vi "awg_memReplay.vi"(6 "reset":bool, 7 "memSelector":refnum<k21>, 9 "periodic":bool, 10 "clocks":T2, 11 "output":bool) -> (0 "pixelPulse":bool, 1 "outputValid":bool, 3 "interpOutput":fxp<+/-,19,2>, 4 "debug":T1, 5 "replayDone":bool)   [LabVIEW 2016]
panel:
  # "Arbitrary Waveform Generator"
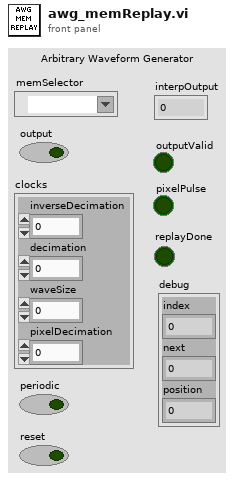
[diagram p1: front panel]
types:
  T1 = cluster{"index":u16, "next":u16, "position":fxp<+,22,0>}
  T2 = cluster{"inverseDecimation":fxp<+,22,0>, "decimation":u16, "waveSize":u16, "pixelDecimation":u16}
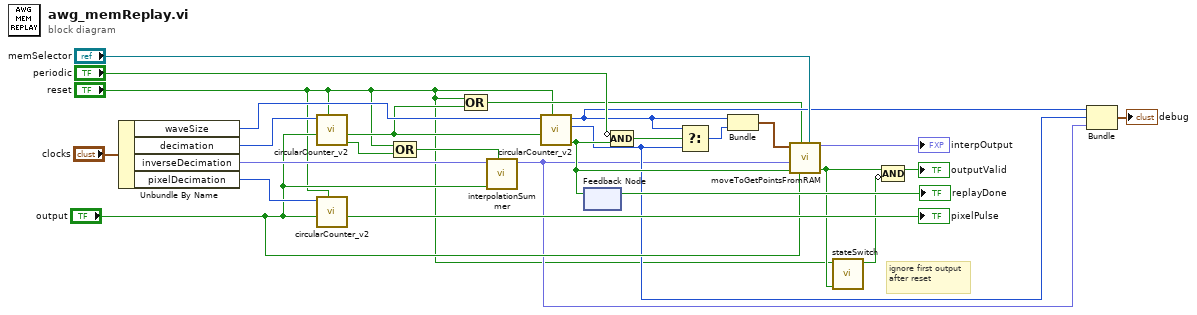
[diagram p0: block diagram]
diagram:
  # "ignore first output after reset"
  n1 = Unbundle By Name("clocks") -> ("waveSize"=w16:u16, "decimation"=w21:u16, "inverseDecimation"=w22:fxp<+,22,0>, "pixelDecimation"=w26:u16)
  n2 = call "circularCounter_v2.vi"("reset"="reset", "doStep"="output", "maxCount"=w21) -> ("maxReached"=w7:bool, "maxPulse"=w6:bool)  [unwired: 5 in, 2 out]
  n3 = call "circularCounter_v2.vi"("reset"="reset", "doStep"="output", "maxCount"=w26) -> ("maxPulse"=→"pixelPulse":bool)  [unwired: 5 in, 3 out]
  n4 = Compound Arithmetic op=OR("reset", w7) -> (w8:bool)
  n5 = Compound Arithmetic op=OR("reset", w6) -> (w5:bool)
  n6 = call "interpolationSummer.vi"("reset"=w8, "doStep"="output", "upStep"=w22) -> ("position"=w10:fxp<+,22,0>)  [unwired: 8 in]
  n7 = call "circularCounter_v2.vi"("reset"="reset", "doStep"=w6, "maxCount"=w16) -> ("maxReached"=w14:bool, "next"=w11:u16, "index"=w12:u16)  [unwired: 5 in, 1 out]
  n8 = feedback-in #1(w14) -> ()
  n9 = feedback #1() -> (→"replayDone":bool)  [unwired: 1 in]
  n10 = Compound Arithmetic op=AND(invert "periodic", w14) -> (w24:bool)
  n11 = Select(t=w12, s=w24, f=w11) -> (s? t:f=w25:u16)
  n12 = Bundle("index"=w12, "next"=w25) -> (w18:cluster{"index":u16, "next":u16})  [unwired: 1 in]
  n13 = call "moveToGetPointsFromRAM.vi"("Memory In"="memSelector", "inputValid"="output", "reset"=w5, "maxReached"=w14, "interpPosition"=w10, "adresses"=w18) -> ("outputValid"=w4:bool, "interpOutput"=→"interpOutput":fxp<+/-,19,2>)  [unwired: 4 in]
  n14 = call "stateSwitch.vi"("disable"=w4, "enable"="reset") -> ("state"=w2:bool)  [unwired: 9 in]
  n15 = Compound Arithmetic op=AND(w4, invert w2) -> (→"outputValid":bool)
  n16 = Bundle("index"=w12, "next"=w11, "position"=w10) -> (→"debug":T1)  [unwired: 1 in]
